vi "Increment_Version_Number.vi"(8 "error in (no error)":errorcluster, 11 "AB_Build in":refnum<class "AB_Build.lvclass">) -> (0 "error out":errorcluster, 3 "AB_Build out":refnum<class "AB_Build.lvclass">)   [LabVIEW 2020, in "AB_Build.lvclass"]
uses:
  <vilib>/AppBuilder/AB_Classes/Build/AB_Build.lvclass
  <vilib>/AppBuilder/AB_Classes/Build/AB_Build.lvclass/AB_Build.ctl
  <vilib>/AppBuilder/RW_Project/AB_RW_Project_PropBag_Action.ctl
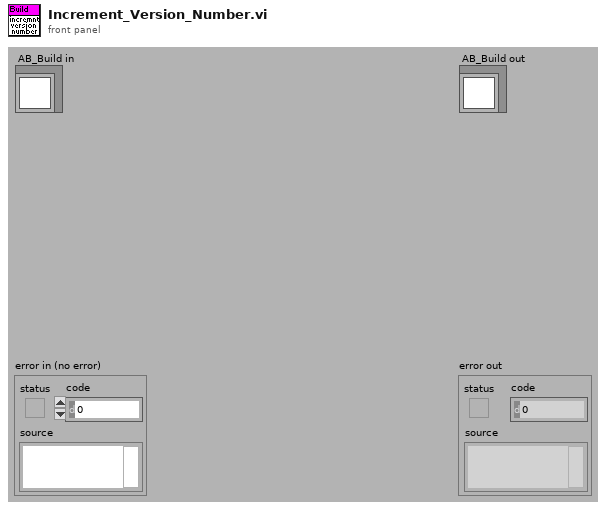
[diagram p1: front panel]
types:
  T1 = typedef "AB_RW_Project_PropBag_Action.ctl" = enum16{"read", "write", "clear", "readPrevious", "writePrevious", "clearPrevious"}
  T2 = typedef "ItemRef.ctl" = u64
  T3 = typedef "AB_RW_Project_Build_Data.ctl" = cluster{"buildSpecName":string, "buildSpecDescription":string, "excludeTypedefs":bool, "excludePolymorphicVIs":bool, "excludeLibraryItems":bool, "modifyLibraryFile":bool, "defaultLanguage":string, "supportedLanguages":string[], "excludedDirectories":path[], "userLog_Path":path, "preActionVIID":string, "postActionVIID":string, "localDest_Path":path, "targetDest_Path":path, "removeVIObject":u16, "previewCache_ID":string, "buildCache_ID":string, "excludeInlineSubVIs":bool, "bldVersion":cluster{"major":u16, "minor":u16, "patch":u16, "build":u16}, "autoIncrement":bool, "excludeDependentPPLs":bool, "excludeDependentDLLs":bool}
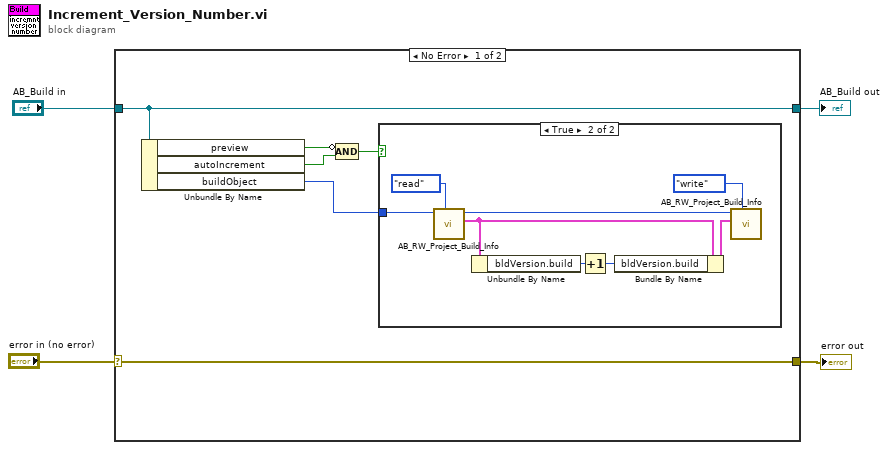
[diagram p0: block diagram]
diagram:
  n1 = case shown="No Error" "error in (no error)" {
    selector: "error in (no error)" -> [w10 w20]
    tunnel: [w10 w20] -> w3
    tunnel: [w9 w19] -> w1
    tunnel: "AB_Build in" -> [w9 w19]
    frame No Error {
      n2 = Unbundle By Name(w9) -> ("preview"=w7:bool, "autoIncrement"=w6:bool, "buildObject"=w8:T2)
      n3 = Compound Arithmetic op=AND(invert w7, w6) -> (w5:bool)
      n4 = case shown="True" w5 {
        tunnel: w8 -> [_ w17]
        frame False {
        }
        frame True {
          n5 = call <vilib>:"AB_RW_Project_Build_Info.vi"("action"=AB_RW_Project_PropBag_Action."read", "Object In"=w17) -> ("buildInfo out"=w14:T3, "Object Out"=w15:T2)  [unwired: 7 in, 1 out]
          n6 = Unbundle By Name(w14) -> ("bldVersion.build"=w13:u16)
          n7 = Increment(x=w13) -> (x+1=w12:u16)
          n8 = Bundle By Name(cluster=w14, "bldVersion.build"=w12) -> (w11:T3)
          n9 = call <vilib>:"AB_RW_Project_Build_Info.vi"("action"=AB_RW_Project_PropBag_Action."write", "buildInfo in"=w11, "Object In"=w15) -> ()  [unwired: 6 in, 3 out]
        }
      }
    }
    frame Error {
    }
  }
  "error out" <- w3
  "AB_Build out" <- w1
